vi "Logger.Variant.Read.Old.vi"(8 "error in (no error)":errorcluster, 11 "VariantSets in":T2={"State"=enum."Init", "ImgPath"=path "", "WabcoPlate"="", "WabcoProduct"="", "ClientProduct"="", "ClientPlate"="", "TotalQuantity"=0, "OrderQuantity"=0, "Serial"=0, "Wabco"={"LaserJob"="", "AdditionalTxt"="037", "FactoryCode"="", "RevID"=0, "ForkID"=0, "FailuresLimit"=0, "GlobalCnt"=0, "CheckDM"=FALSE, "SerialFormat"=enum."6 dig", "CoordA"={"X"=0.0, "Y"=0.0, "Angle"=0.0}, "CoordB"={"X"=0.0, "Y"=0.0, "Angle"=0.0}, "DMCconfig"=0}, "Client"={"LaserJob"="", "AdditionalTxt"="", "FactoryCode"="037", "RevID"=0, "ForkID"=0, "FailuresLimit"=0, "GlobalCnt"=0, "CheckDM"=FALSE, "SerialFormat"=enum."6 dig", "CoordA"={"X"=0.0, "Y"=0.0, "Angle"=0.0}, "CoordB"={"X"=0.0, "Y"=0.0, "Angle"=0.0}, "DMCconfig"=0}}) -> (0 "error out":errorcluster, 1 "ClientPlateImg":picture, 2 "WabcoPlateImg":picture, 3 "VariantSets out":T2={"State"=enum."Init", "ImgPath"=path "", "WabcoPlate"="", "WabcoProduct"="", "ClientProduct"="", "ClientPlate"="", "TotalQuantity"=0, "OrderQuantity"=0, "Serial"=0, "Wabco"={"LaserJob"="", "AdditionalTxt"="037", "FactoryCode"="", "RevID"=0, "ForkID"=0, "FailuresLimit"=0, "GlobalCnt"=0, "CheckDM"=FALSE, "SerialFormat"=enum."6 dig", "CoordA"={"X"=0.0, "Y"=0.0, "Angle"=0.0}, "CoordB"={"X"=0.0, "Y"=0.0, "Angle"=0.0}, "DMCconfig"=0}, "Client"={"LaserJob"="", "AdditionalTxt"="", "FactoryCode"="037", "RevID"=0, "ForkID"=0, "FailuresLimit"=0, "GlobalCnt"=0, "CheckDM"=FALSE, "SerialFormat"=enum."6 dig", "CoordA"={"X"=0.0, "Y"=0.0, "Angle"=0.0}, "CoordB"={"X"=0.0, "Y"=0.0, "Angle"=0.0}, "DMCconfig"=0}}, 5 "OrdersTableIdx":i32, 7 "OrdersTable":string[][](array[string]))   [LabVIEW 2016]
uses:
  Logger.Variant.Sets.ctl
  Station/Station.Changeover.State.vi
  Station/Station.Plate.Properties.ctl
  Sequence/Sequence.Code.SerialFormat.ctl
  Drivers/V7310/LowLevel/V7310.Job.Sets.ctl
  Global/ApplicationGlobal.vi
  Drivers/V7310/LowLevel/V7310.Global.vi
panel:
  in  "SerialFormat":T1
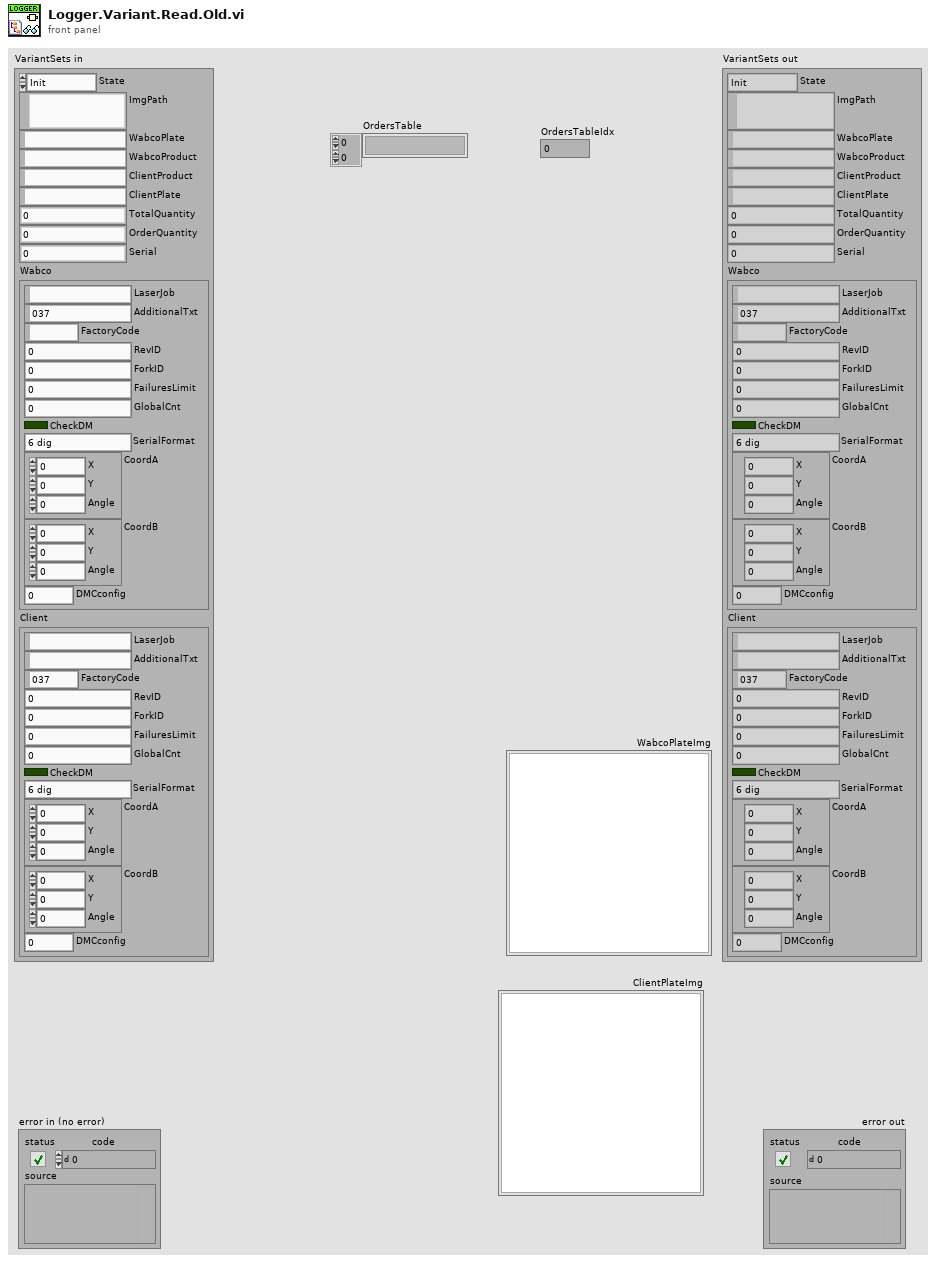
[diagram p1: front panel]
types:
  T1 = typedef "Sequence.Code.SerialFormat.ctl" = enum8{"", "6 dig", "7 dig"}
  T2 = typedef "Logger.Variant.Sets.ctl" = cluster{"State":T3, "ImgPath":path, "WabcoPlate":string, "WabcoProduct":string, "ClientProduct":string, "ClientPlate":string, "TotalQuantity":u16, "OrderQuantity":u16, "Serial":i32, "Wabco":T4, "Client":T4}
  T3 = typedef "Station.Changeover.State.vi" = enum16{"Init", "Scaning", "NOK", "Wait for ack", "Ready"}
  T4 = typedef "Station.Plate.Properties.ctl" = cluster{"LaserJob":string, "AdditionalTxt":string, "FactoryCode":string, "RevID":u8, "ForkID":u8, "FailuresLimit":u16, "GlobalCnt":i32, "CheckDM":bool, "SerialFormat":T1, "CoordA":T5, "CoordB":T5, "DMCconfig":i32}
  T5 = typedef "V7310.Job.Sets.ctl" = cluster{"X":dbl, "Y":dbl, "Angle":dbl}
  T6 = cluster{"WabcoPlate":string, "WabcoProduct":string, "ClientProduct":string, "ClientPlate":string}
  T7 = typedef "imagedata.ctl" = cluster{"image type":i32, "image depth":i32, "image":u8[], "mask":u8[], "colors":u32[], "Rectangle":cluster{"left":i16, "top":i16, "right":i16, "bottom":i16}}
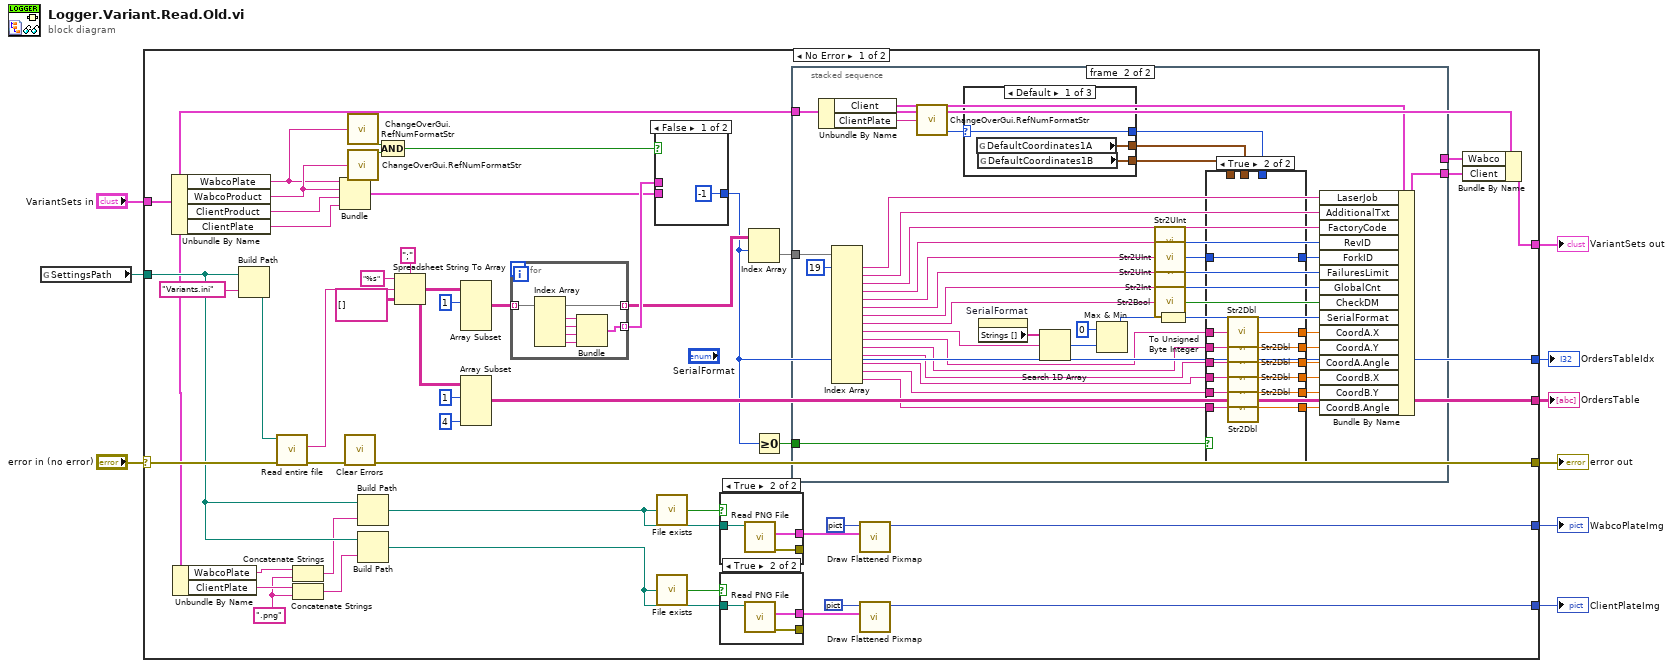
[diagram p0: block diagram]
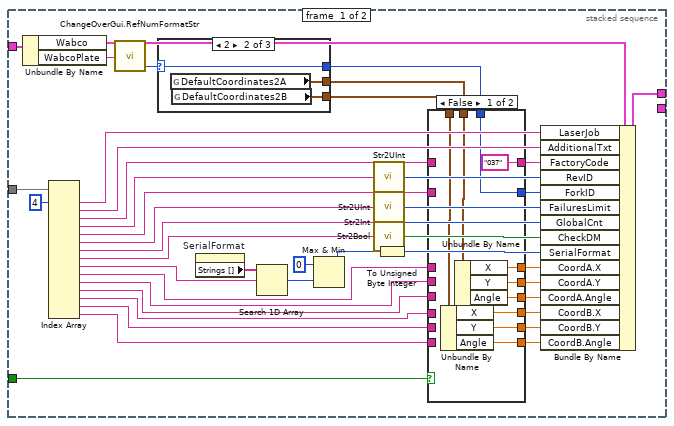
[diagram p2: hidden frame]
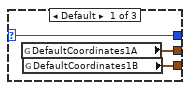
[diagram p3: hidden frame]
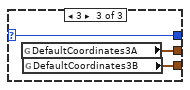
[diagram p4: hidden frame]
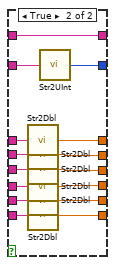
[diagram p5: hidden frame]
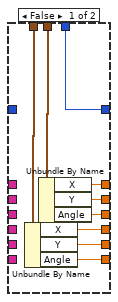
[diagram p6: hidden frame]
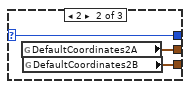
[diagram p7: hidden frame]
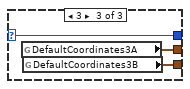
[diagram p8: hidden frame]
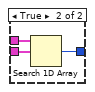
[diagram p9: hidden frame]
diagram:
  n1 = global read "ApplicationGlobal.vi" "SettingsPath"() -> (w7:path)
  n2 = case shown="No Error" "error in (no error)" {
    selector: "error in (no error)" -> [w56 w225]
    tunnel: [w24 w225] -> w8
    tunnel: w7 -> [w47 _]
    tunnel: [w20 _] -> w5
    tunnel: [w57 _] -> w6
    tunnel: "VariantSets in" -> [w12 _]
    tunnel: [w36 _] -> w3
    tunnel: [w13 _] -> w2
    tunnel: [w11 _] -> w1
    frame No Error {
      w43 = ".png" ("string")
      n3 = Unbundle By Name(w12) -> ("WabcoPlate"=w26:string, "WabcoProduct"=w27:string, "ClientProduct"=w34:string, "ClientPlate"=w17:string)
      n4 = Unbundle By Name(w12) -> ("WabcoPlate"=w44:string, "ClientPlate"=w46:string)
      n5 = Build Path(base path=w47, name or relative path="Variants.ini" ("format string")) -> (appended path=w52:path)
      n6 = call "Read entire file.vi"("error in"=w56, "file"=w52) -> ("error out"=w31:errorcluster, "contents"=w51:string)  [unwired: 4 in]
      n7 = Concatenate Strings(w44, w43) -> (w42:string)
      n8 = Concatenate Strings(w46, w43) -> (w45:string)
      n9 = Bundle("WabcoPlate"=w26, "WabcoProduct"=w27, "ClientProduct"=w34, "ClientPlate"=w17) -> (w32:T6)  [unwired: 1 in]
      n10 = call <vilib>:"Clear Errors.vi"("error in (no error)"=w31) -> ("error out"=w24:errorcluster)  [unwired: 5 in, 1 out]
      n11 = call "ChangeOverGui.RefNumFormatStr.vi"("RefNum in"=w26) -> ("RefNum format ok?"=w29:bool)  [unwired: 2 out]
      n12 = call "ChangeOverGui.RefNumFormatStr.vi"("RefNum in"=w27) -> ("RefNum format ok?"=w28:bool)  [unwired: 2 out]
      n13 = Build Path(base path=w47, name or relative path=w42) -> (appended path=w41:path)
      n14 = Build Path(base path=w47, name or relative path=w45) -> (appended path=w37:path)
      n15 = Compound Arithmetic op=AND(w29, w28) -> (w25:bool)
      n16 = Spreadsheet String To Array(delimiter (Tab)=";", format string="%s", spreadsheet string=w51, array type (2D Dbl)=string[][] []) -> (array=w16:string[][])
      n17 = Array Subset(array=w16, index (row)=1 ("index")) -> (w23:string[][])  [unwired: 3 in]
      n18 = Array Subset(array=w16, index (row)=1 ("index"), length (col)=4 ("length")) -> (w13:string[][])  [unwired: 2 in]
      n19 = for {
        tunnel: w23 -> [w210] mode=indexing
        tunnel: [w211] -> w33 mode=indexing
        tunnel: [w210] -> w22 mode=indexing
        n20 = Index Array(array=w210) -> (element #1=w214:string, element #2=w213:string, element #3=w212:string, element #4=w209:string)  [unwired: 4 in]
        n21 = Bundle(w214, w213, w212, w209) -> (w211:cluster{string, string, string, string})  [unwired: 1 in]
      }
      n22 = case shown="False" w25 {
        tunnel: w33 -> [_ w218]
        tunnel: w32 -> [_ w217]
        tunnel: [-1 ("index of element") w216] -> w11
        frame False {
        }
        frame True {
          n23 = Search 1D Array(1D array=w218, element=w217) -> (index of element=w216:i32)  [unwired: 1 in]
        }
      }
      n24 = call "File exists.vi"("file path"=w41) -> ("exists?"=w55:bool)  [unwired: 4 in]
      n25 = call "File exists.vi"("file path"=w37) -> ("exists?"=w38:bool)  [unwired: 4 in]
      n26 = case shown="True" w55 {
        tunnel: w41 -> [_ w224]
        tunnel: [_ w223] -> w53
        tunnel: [_ w222] -> _
        frame False {
        }
        frame True {
          n27 = call <vilib>:"Read PNG File.vi"("path to PNG file"=w224) -> ("error out"=w222:errorcluster, "image data"=w223:T7)  [unwired: 8 in, 1 out]
        }
      }
      n28 = case shown="True" w38 {
        tunnel: w37 -> [_ w221]
        tunnel: [_ w220] -> w40
        tunnel: [_ w219] -> _
        frame False {
        }
        frame True {
          n29 = call <vilib>:"Read PNG File.vi"("path to PNG file"=w221) -> ("error out"=w219:errorcluster, "image data"=w220:T7)  [unwired: 8 in, 1 out]
        }
      }
      n30 = Index Array(array=w22, index (row)=w11) -> (element=w21:string[])  [unwired: 1 in]
      n31 = Greater Or Equal To 0?(x=w11) -> (x >= 0?=w10:bool)
      n32 = stacked-sequence {
        tunnel: w21 -> [w98 w175]
        tunnel: w12 -> [w68 w155]
        tunnel: [w96 _] -> w19
        tunnel: [_ w156] -> w18
        tunnel: w10 -> [w67 w152]
        frame #0 {
          n33 = Unbundle By Name(w68) -> ("Wabco"=w100:T4, "WabcoPlate"=w66:string)
          n34 = Index Array(array=w98, index #1=4 ("index")) -> (element #1=w97:string, element #2=w95:string, element #3=w62:string, element #4=w93:string, element #5=w58:string, element #6=w91:string, element #7=w89:string, element #8=w87:string, element #9=w75:string, element #10=w74:string, element #11=w73:string, element #12=w72:string, element #13=w71:string, element #14=w70:string, element #15=w69:string)  [unwired: 14 in]
          n35 = call "ChangeOverGui.RefNumFormatStr.vi"("RefNum in"=w66) -> ("Idx"=w65:i32)  [unwired: 2 out]
          n36 = case shown="2" w65 {
            selector: w65 -> [w101 w104 w107]
            tunnel: [w103 w106 w109] -> w64
            tunnel: [w102 w105 w108] -> w63
            tunnel: [w101 w104 w107] -> w60
            frame Default {
              n37 = global read "V7310.Global.vi" "DefaultCoordinates1A"() -> (w103:T5)
              n38 = global read "V7310.Global.vi" "DefaultCoordinates1B"() -> (w102:T5)
            }
            frame 2 {
              n39 = global read "V7310.Global.vi" "DefaultCoordinates2A"() -> (w106:T5)
              n40 = global read "V7310.Global.vi" "DefaultCoordinates2B"() -> (w105:T5)
            }
            frame 3 {
              n41 = global read "V7310.Global.vi" "DefaultCoordinates3A"() -> (w109:T5)
              n42 = global read "V7310.Global.vi" "DefaultCoordinates3B"() -> (w108:T5)
            }
          }
          n43 = property on="SerialFormat" class="Enum (strict)"() -> ("Strings []"=w86:string[])  [unwired: 2 in, 2 out]
          n44 = Search 1D Array(1D array=w86, element=w75) -> (index of element=w85:i32)  [unwired: 1 in]
          n45 = Max & Min(x=0, y=w85) -> (max(x,y)=w82:i32)  [unwired: 1 out]
          n46 = call "Str2UInt.vi"("string"=w93) -> ("Numeric"=w94:u32)
          n47 = call "Str2UInt.vi"("string"=w91) -> ("Numeric"=w92:u32)
          n48 = call "Str2Int.vi"("string"=w89) -> ("Numeric"=w90:i32)
          n49 = call "Str2Bool.vi"("string"=w87) -> ("Boolean"=w88:bool)
          n50 = To Unsigned Byte Integer(number=w82) -> (unsigned 8bit integer=w83:u8)
          n51 = case shown="False" w67 {
            tunnel: [w118 w134] -> w81
            tunnel: [w117 w133] -> w80
            tunnel: [w116 w132] -> w79
            tunnel: [w114 w131] -> w78
            tunnel: [w113 w130] -> w77
            tunnel: [w112 w129] -> w76
            tunnel: w74 -> [_ w128]
            tunnel: w73 -> [_ w127]
            tunnel: w72 -> [_ w126]
            tunnel: w71 -> [_ w125]
            tunnel: w70 -> [_ w124]
            tunnel: w69 -> [_ w123]
            tunnel: w64 -> [w119 _]
            tunnel: w63 -> [w115 _]
            tunnel: w62 -> [_ w122]
            tunnel: ["037" w122] -> w61
            tunnel: w60 -> [w110 _]
            tunnel: [w110 w120] -> w59
            tunnel: w58 -> [_ w121]
            frame False {
              n52 = Unbundle By Name(w115) -> ("X"=w114:dbl, "Y"=w113:dbl, "Angle"=w112:dbl)
              n53 = Unbundle By Name(w119) -> ("X"=w118:dbl, "Y"=w117:dbl, "Angle"=w116:dbl)
            }
            frame True {
              n54 = call "Str2Dbl.vi"("string"=w128) -> ("Numeric"=w134:dbl)
              n55 = call "Str2Dbl.vi"("string"=w127) -> ("Numeric"=w133:dbl)
              n56 = call "Str2Dbl.vi"("string"=w126) -> ("Numeric"=w132:dbl)
              n57 = call "Str2Dbl.vi"("string"=w125) -> ("Numeric"=w131:dbl)
              n58 = call "Str2Dbl.vi"("string"=w124) -> ("Numeric"=w130:dbl)
              n59 = call "Str2Dbl.vi"("string"=w123) -> ("Numeric"=w129:dbl)
              n60 = call "Str2UInt.vi"("string"=w121) -> ("Numeric"=w120:u32)
            }
          }
          n61 = Bundle By Name(cluster=w100, "LaserJob"=w97, "AdditionalTxt"=w95, "FactoryCode"=w61, "RevID"=w94, "ForkID"=w59, "FailuresLimit"=w92, "GlobalCnt"=w90, "CheckDM"=w88, "SerialFormat"=w83, "CoordA.X"=w81, "CoordA.Y"=w80, "CoordA.Angle"=w79, "CoordB.X"=w78, "CoordB.Y"=w77, "CoordB.Angle"=w76) -> (w96:T4)
        }
        frame #1 {
          n62 = Unbundle By Name(w155) -> ("Client"=w177:T4, "ClientPlate"=w153:string)
          n63 = Index Array(array=w175, index #1=19 ("index")) -> (element #1=w174:string, element #2=w173:string, element #3=w172:string, element #4=w170:string, element #5=w169:string, element #6=w167:string, element #7=w165:string, element #8=w163:string, element #9=w157:string, element #10=w149:string, element #11=w148:string, element #12=w147:string, element #13=w150:string, element #14=w151:string, element #15=w146:string)  [unwired: 14 in]
          n64 = call "ChangeOverGui.RefNumFormatStr.vi"("RefNum in"=w153) -> ("Idx"=w154:i32)  [unwired: 2 out]
          n65 = case shown="Default" w154 {
            selector: w154 -> [w200 w203 w206]
            tunnel: [w202 w205 w208] -> w145
            tunnel: [w201 w204 w207] -> w144
            tunnel: [w200 w203 w206] -> w136
            frame Default {
              n66 = global read "V7310.Global.vi" "DefaultCoordinates1A"() -> (w202:T5)
              n67 = global read "V7310.Global.vi" "DefaultCoordinates1B"() -> (w201:T5)
            }
            frame 2 {
              n68 = global read "V7310.Global.vi" "DefaultCoordinates2A"() -> (w205:T5)
              n69 = global read "V7310.Global.vi" "DefaultCoordinates2B"() -> (w204:T5)
            }
            frame 3 {
              n70 = global read "V7310.Global.vi" "DefaultCoordinates3A"() -> (w208:T5)
              n71 = global read "V7310.Global.vi" "DefaultCoordinates3B"() -> (w207:T5)
            }
          }
          n72 = property on="SerialFormat" class="Enum (strict)"() -> ("Strings []"=w162:string[])  [unwired: 2 in, 2 out]
          n73 = Search 1D Array(1D array=w162, element=w157) -> (index of element=w161:i32)  [unwired: 1 in]
          n74 = Max & Min(x=0, y=w161) -> (max(x,y)=w158:i32)  [unwired: 1 out]
          n75 = call "Str2UInt.vi"("string"=w170) -> ("Numeric"=w171:u32)
          n76 = call "Str2UInt.vi"("string"=w169) -> ("Numeric"=w135:u32)
          n77 = call "Str2UInt.vi"("string"=w167) -> ("Numeric"=w168:u32)
          n78 = call "Str2Int.vi"("string"=w165) -> ("Numeric"=w166:i32)
          n79 = call "Str2Bool.vi"("string"=w163) -> ("Boolean"=w164:bool)
          n80 = To Unsigned Byte Integer(number=w158) -> (unsigned 8bit integer=w159:u8)
          n81 = case shown="True" w152 {
            tunnel: [w185 w199] -> w143
            tunnel: [w184 w198] -> w142
            tunnel: [w183 w197] -> w141
            tunnel: [w181 w196] -> w140
            tunnel: [w180 w195] -> w139
            tunnel: [w179 w194] -> w138
            tunnel: w145 -> [w186 _]
            tunnel: w144 -> [w182 _]
            tunnel: w151 -> [_ w193]
            tunnel: w150 -> [_ w192]
            tunnel: w149 -> [_ w191]
            tunnel: w148 -> [_ w190]
            tunnel: w147 -> [_ w189]
            tunnel: w146 -> [_ w188]
            tunnel: [w178 w187] -> w137
            tunnel: w136 -> [w178 _]
            tunnel: w135 -> [_ w187]
            frame False {
              n82 = Unbundle By Name(w182) -> ("X"=w181:dbl, "Y"=w180:dbl, "Angle"=w179:dbl)
              n83 = Unbundle By Name(w186) -> ("X"=w185:dbl, "Y"=w184:dbl, "Angle"=w183:dbl)
            }
            frame True {
              n84 = call "Str2Dbl.vi"("string"=w191) -> ("Numeric"=w199:dbl)
              n85 = call "Str2Dbl.vi"("string"=w190) -> ("Numeric"=w198:dbl)
              n86 = call "Str2Dbl.vi"("string"=w189) -> ("Numeric"=w197:dbl)
              n87 = call "Str2Dbl.vi"("string"=w192) -> ("Numeric"=w196:dbl)
              n88 = call "Str2Dbl.vi"("string"=w193) -> ("Numeric"=w195:dbl)
              n89 = call "Str2Dbl.vi"("string"=w188) -> ("Numeric"=w194:dbl)
            }
          }
          n90 = Bundle By Name(cluster=w177, "LaserJob"=w174, "AdditionalTxt"=w173, "FactoryCode"=w172, "RevID"=w171, "ForkID"=w137, "FailuresLimit"=w168, "GlobalCnt"=w166, "CheckDM"=w164, "SerialFormat"=w159, "CoordA.X"=w143, "CoordA.Y"=w142, "CoordA.Angle"=w141, "CoordB.X"=w140, "CoordB.Y"=w139, "CoordB.Angle"=w138) -> (w156:T4)
        }
      }
      n91 = call <vilib>:"Draw Flattened Pixmap.vi"("image data"=w53, "picture"=picture data[5B]) -> ("new picture"=w57:picture)  [unwired: 7 in]
      n92 = call <vilib>:"Draw Flattened Pixmap.vi"("image data"=w40, "picture"=picture data[5B]) -> ("new picture"=w36:picture)  [unwired: 7 in]
      n93 = Bundle By Name(cluster=w12, "Wabco"=w19, "Client"=w18) -> (w20:T2)
    }
    frame Error {
    }
  }
  "error out" <- w8
  "WabcoPlateImg" <- w6
  "VariantSets out" <- w5
  "ClientPlateImg" <- w3
  "OrdersTable" <- w2
  "OrdersTableIdx" <- w1
